vi "Get LV Class Default Value By Name - NONUI.vi"(8 "error in (no error)":errorcluster, 10 "apprefnum":u32, 11 "class name":string) -> (0 "error out":errorcluster, 3 "object":refnum<class>)   [LabVIEW 2019, in "IncrementMutationHistory.lvlib" / "VILIB_NONUI.lvlib"]
doc: "Returns the class data for the class whose name you wire to the <B>class name</B> input. If the class is not in memory or is broken, LabVIEW returns an error."
uses:
  VILIB_NONUI.lvlib
panel:
  in  "Empty Name":string="<Empty Name>"
  in  "error message":string="LabVIEW attempted to find the class with this name:"
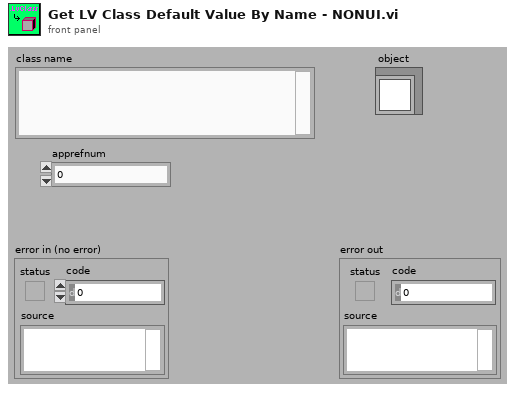
[diagram p1: front panel]
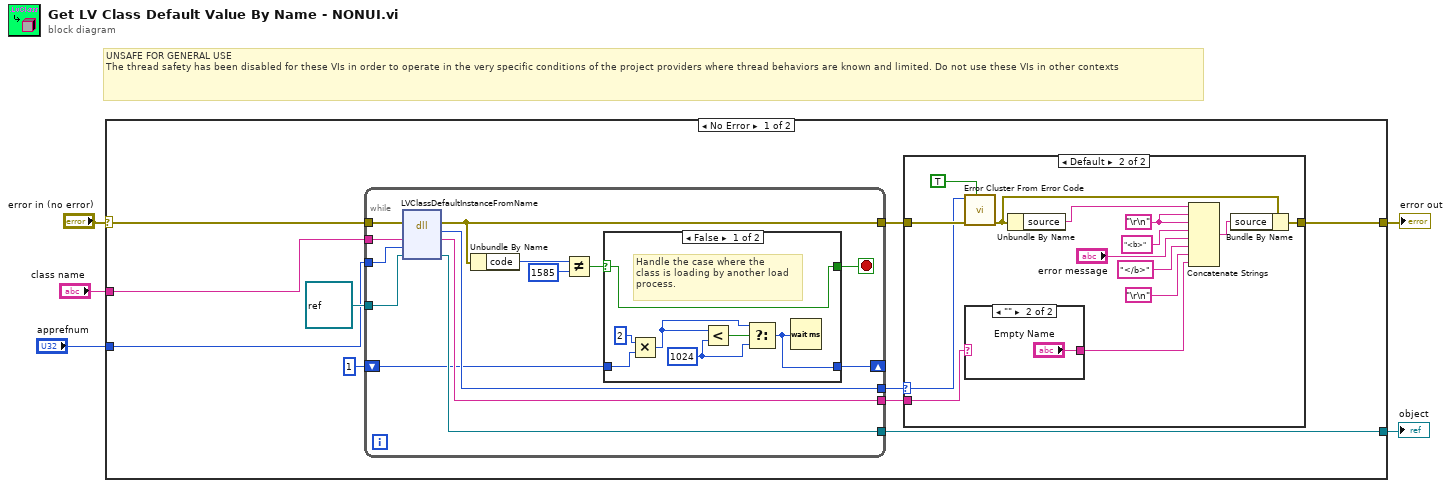
[diagram p0: block diagram]
diagram:
  # "UNSAFE FOR GENERAL USE\nThe thread safety has been disabled for these VIs in order to operate in the very specific conditions of the project providers where thread behaviors are known and limited. Do not use these VIs in other contexts"
  n1 = case shown="No Error" "error in (no error)" {
    selector: "error in (no error)" -> [w7 w56]
    tunnel: [w6 w56] -> w5
    tunnel: [w15 _] -> w3
    tunnel: "class name" -> [w9 _]
    tunnel: "apprefnum" -> [w8 _]
    frame No Error {
      n2 = while {
        tunnel: w7 -> [w29]
        tunnel: [w28] -> w15
        tunnel: refnum<class> refnum ("classData") -> [w27]
        tunnel: w8 -> [w26]
        tunnel: [w25] -> w13
        tunnel: w9 -> [w24]
        tunnel: [w23] -> w12
        tunnel: [w22] -> w11
        shift-right: [w17] -> _
        shift-left: u32 1 -> [w16]
        stop <- w18 stop-if-true
        n3 = dll-call lib="LabVIEW" fn="LVClassDefaultInstanceFromName"(error in=w29, "name"=w24, "appRef"=w26, "classData"=w27) -> (error out=w22:errorcluster, "err"=w25:i32, "name"=w23:string, "classData"=w28:refnum<class>)  [unwired: 3 in, 1 out]
        n4 = Unbundle By Name(w22) -> ("code"=w21:i32)
        n5 = Not Equal?(x=w21, y=1585) -> (x != y?=w19:bool)
        n6 = case shown="False" w19 {
          selector: w19 -> [w36 w38]
          tunnel: [w36 w38] -> w18
          tunnel: w16 -> [w30 w37]
          tunnel: [w31 w37] -> w17
          frame False {
            w35 = u32 1024 ("unsigned 32bit integer")
            # "Handle the case where the \nclass is loading by another load\nprocess."
            n7 = Multiply(x=u32 2 ("y"), y=w30) -> (x*y=w32:u32)
            n8 = Less?(x=w32, y=w35) -> (x < y?=w34:bool)
            n9 = Select(t=w32, s=w34, f=w35) -> (s? t:f=w31:u32)
            n10 = Wait (ms)(milliseconds to wait=w31) -> ()  [unwired: 1 out]
          }
          frame True {
          }
        }
      }
      n11 = case shown="Default" w13 {
        selector: w13 -> [_ w51]
        tunnel: w12 -> [_ w40]
        tunnel: [w39 w50] -> w6
        tunnel: w11 -> [w39 w52]
        frame 0 {
        }
        frame Default {
          w47 = "\r\n"
          n12 = call <vilib>:"Error Cluster From Error Code.vi"("show call chain? (False)"=TRUE, "error in (no error)"=w52, "error code (0)"=w51) -> ("error out"=w49:errorcluster)  [unwired: 6 out]
          n13 = case shown="\"\"" w40 {
            selector: w40 -> [w54 _]
            tunnel: [w54 "Empty Name"] -> w41
            frame Default {
            }
            frame "" {
            }
          }
          n14 = Unbundle By Name(w49) -> ("source"=w46:string)
          n15 = Concatenate Strings(w46, w47, w47, "<b>", "error message", "</b>", "\r\n", w41) -> (w48:string)
          n16 = Bundle By Name(cluster=w49, "source"=w48) -> (w50:errorcluster)
        }
      }
    }
    frame Error {
    }
  }
  "error out" <- w5
  "object" <- w3
